vi "program glowny.vi"() -> ()   [LabVIEW 2014]
doc: "Program przeprowadza symulację sklepu, podlicza statystyki np. zarobki. Tablice liczba kas i Natężenie ustawiają odpowiednio liczbę otwartych kas w poszczególnych godzinach oraz wartość oczekiwaną liczby klientów w odpowiednich godzinach. Jeżeli klient przychodzi do sklepu i w kolejce stoi już 10 klientów to wychodzi ze sklepu, staje się klientem straconym. Liczby takich klientów przedstawione są na wykresie Straceni klienci. Przycisk clear resetuje statystyki sklepu. Można ustawić pensję pracowników na kasie za godzinę."
uses:
  sklep.ctl
  event.ctl
panel:
  in  "Pensja za godzine":i32
  out "Sklep":T1
  in  "clear Button":bool
  out "liczba klientów":i32[](graph)
  out "zarobek":i32[](graph)
  in  "stop":bool
  in  "simulate Button":bool
  out "Straceni klienci":i32[](graph)
  out "średni czas w kolejce":dbl[](array[numeric])
  in  "Liczba kas":i32[](array[numeric])
  in  "Natężenie(per h)":i32[](array[numeric])
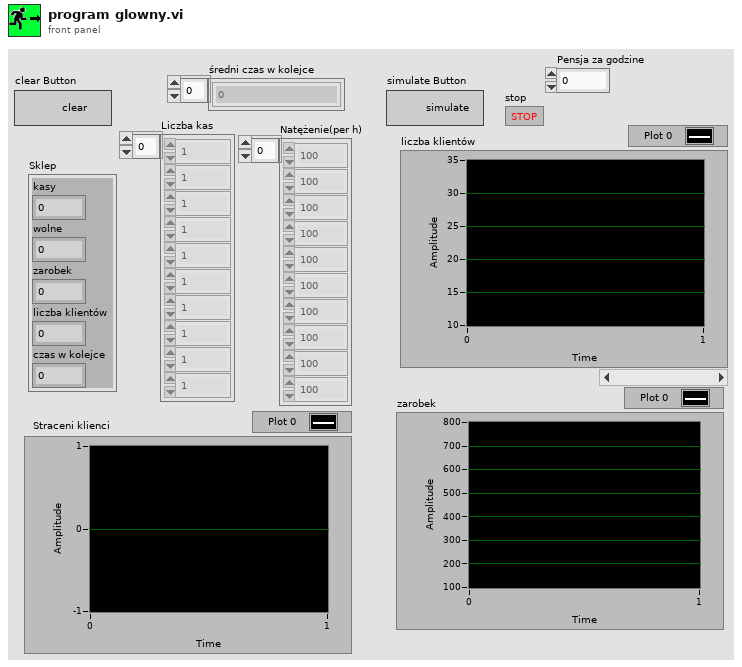
[diagram p1: front panel]
types:
  T1 = typedef "sklep.ctl" = cluster{"kasy":i32, "wolne":i32, "zarobek":i32, "liczba klientów":i32, "czas w kolejce":u64}
  T2 = typedef "event.ctl" = cluster{"czas":u32, "event":enum16{"przyjście klienata", "zwolnienie kasy", "oczekiwanie na klienta", "nowy event"}}
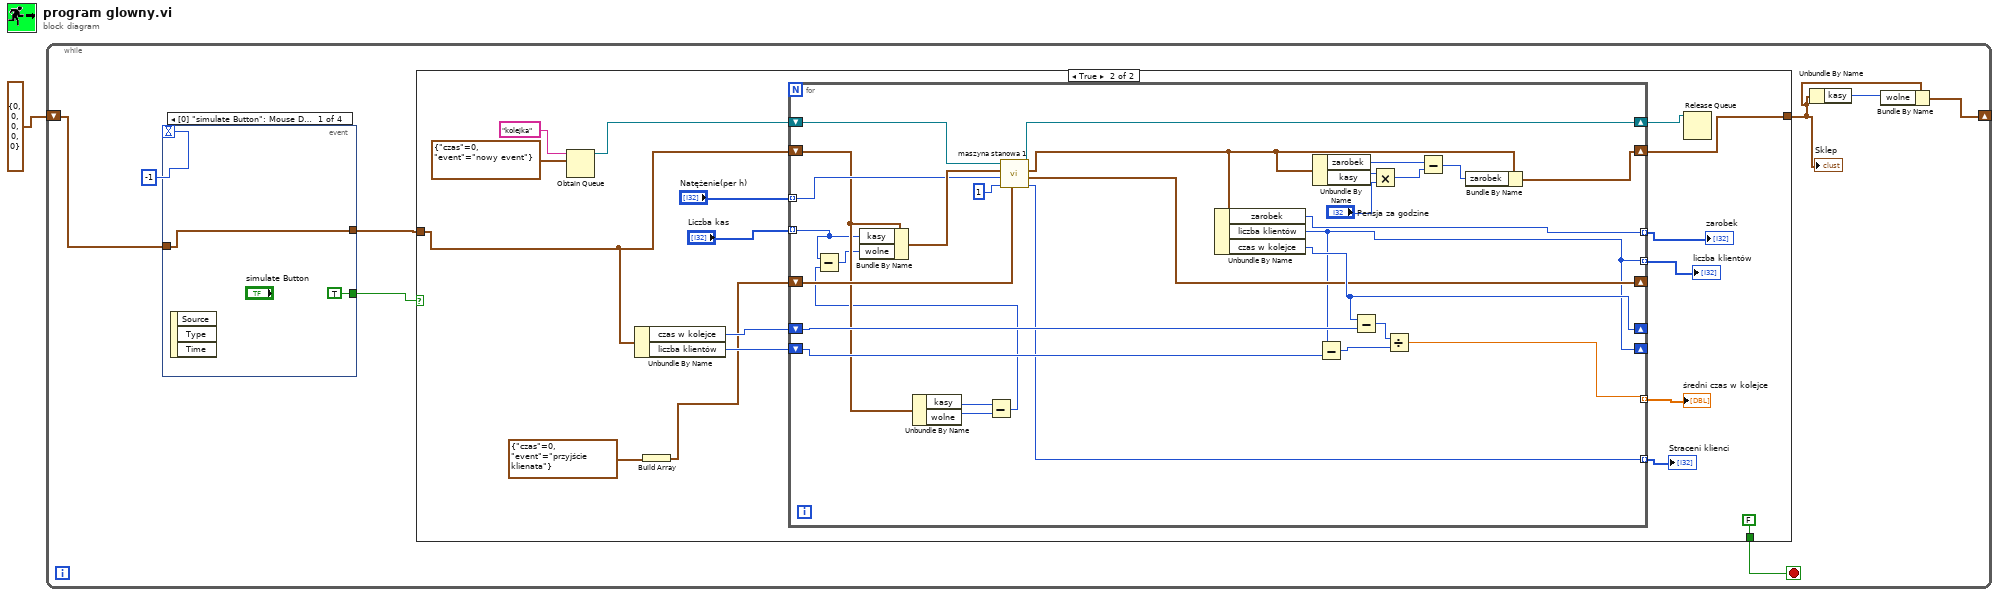
[diagram p0: block diagram]
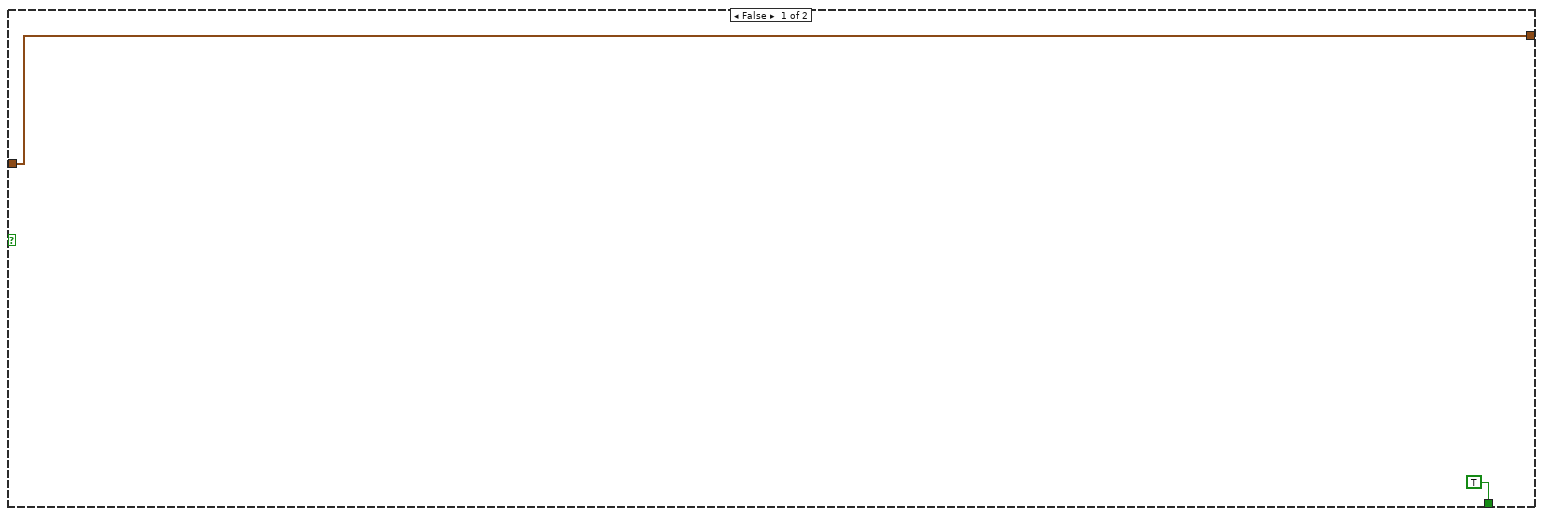
[diagram p2: hidden frame]
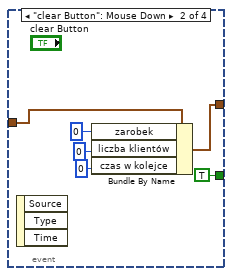
[diagram p3: hidden frame]
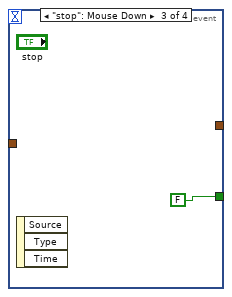
[diagram p4: hidden frame]
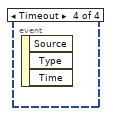
[diagram p5: hidden frame]
diagram:
  n1 = while {
    shift-right: [w5] -> _
    shift-left: T1 {"kasy"=0, "wolne"=0, "zarobek"=0, "liczba klientów"=0, "czas w kolejce"=0} ("Sklep") -> [w3]
    stop <- w7 stop-if-true
    n2 = event shown="[0] \"simulate Button\": Mouse Down" {
      selector: _ -> [_ _ _ _]
      dyn-events: _ -> [_ _ _ _]
      timeout: -1 -> [_ _ _ _]
      tunnel: [TRUE TRUE FALSE _] -> w9
      tunnel: w3 -> [w58 w65 _ _]
      tunnel: [w58 w64 _ _] -> w2
      event "simulate Button": Mouse Down {
        n3 = event-data() -> ()  [unwired: 1 in, 3 out]
      }
      event "clear Button": Mouse Down {
        n4 = event-data() -> ()  [unwired: 1 in, 3 out]
        n5 = Bundle By Name(cluster=w65, "zarobek"=0, "liczba klientów"=0, "czas w kolejce"=u64 0) -> (w64:T1)
      }
      event "stop": Mouse Down {
        n6 = event-data() -> ()  [unwired: 1 in, 3 out]
      }
      event Timeout {
        n7 = event-data() -> ()  [unwired: 1 in, 3 out]
      }
    }
    n8 = case shown="True" w9 {
      tunnel: [TRUE FALSE] -> w7
      tunnel: w2 -> [w10 w13]
      tunnel: [w10 w12] -> w4
      frame False {
      }
      frame True {
        n9 = Obtain Queue(name (unnamed)="kolejka", element data type=T2 {"czas"=0, "event"=enum."nowy event"} ("Cluster")) -> (queue out=w24:refnum<queue>)  [unwired: 3 in, 2 out]
        n10 = Unbundle By Name(w13) -> ("czas w kolejce"=w23:u64, "liczba klientów"=w22:i32)
        n11 = Build Array(T2 {"czas"=0, "event"=enum."przyjście klienata"} ("Cluster")) -> (w19:T2[])
        n12 = for {
          shift-right: [w32] -> w12
          shift-left: w13 -> [w45]
          tunnel: "Liczba kas" -> [w42] mode=indexing
          tunnel: "Natężenie(per h)" -> [w55] mode=indexing
          shift-right: [w52] -> w14
          shift-left: w24 -> [w56]
          shift-right: [w46] -> _
          shift-left: w19 -> [w53]
          shift-right: [w47] -> _
          shift-left: w23 -> [w51]
          shift-right: [w36] -> _
          shift-left: w22 -> [w50]
          tunnel: [w39] -> w21 mode=indexing
          tunnel: [w38] -> w18 mode=indexing
          tunnel: [w37] -> w16 mode=indexing
          tunnel: [w36] -> w15 mode=indexing
          n13 = Unbundle By Name(w45) -> ("kasy"=w44:i32, "wolne"=w43:i32)
          n14 = Subtract(x=w44, y=w43) -> (x-y=w41:i32)
          n15 = Subtract(x=w42, y=w41) -> (x-y=w40:i32)
          n16 = Bundle By Name(cluster=w45, "kasy"=w42, "wolne"=w40) -> (w57:T1)
          n17 = call "maszyna stanowa 1.vi"("Niewykonane eventy in"=w53, "Ile godzin"=1, "Liczba klientów na godzinę"=w55, "Sklep in"=w57, "queue in"=w56) -> ("Straceni klienci"=w38:i32, "Niewykonane eventy out"=w46:T2[], "Sklep out"=w35:T1, "queue out"=w52:refnum<queue>)  [unwired: 3 in]
          n18 = Unbundle By Name(w35) -> ("zarobek"=w37:i32, "liczba klientów"=w36:i32, "czas w kolejce"=w47:u64)
          n19 = Unbundle By Name(w35) -> ("zarobek"=w31:i32, "kasy"=w34:i32)
          n20 = Subtract(x=w36, y=w50) -> (x-y=w48:i32)
          n21 = Subtract(x=w47, y=w51) -> (x-y=w49:u64)
          n22 = Multiply(x=w34, y="Pensja za godzine") -> (x*y=w30:i32)
          n23 = Divide(x=w49, y=w48) -> (x/y=w39:dbl)
          n24 = Subtract(x=w31, y=w30) -> (x-y=w29:i32)
          n25 = Bundle By Name(cluster=w35, "zarobek"=w29) -> (w32:T1)
        }
        "średni czas w kolejce" <- w21
        "Straceni klienci" <- w18
        "zarobek" <- w16
        "liczba klientów" <- w15
        n26 = Release Queue(queue=w14) -> ()  [unwired: 2 in, 3 out]
      }
    }
    "Sklep" <- w4
    n27 = Unbundle By Name(w4) -> ("kasy"=w6:i32)
    n28 = Bundle By Name(cluster=w4, "wolne"=w6) -> (w5:T1)
  }
